vi "FV-resample-pad_data.vi"(11 "output cluster":T1) -> (1 "Array":cluster{"Y":dbl[], "Y":dbl[]}[](array[cluster]), 2 "appended array":waveform(dbl)[](array[waveform]), 3 "output cluster 2":T1)   [LabVIEW 2020, in "FV-file_viewer.lvlib"]
uses:
  FV-file_viewer.lvlib
  FV-splitting_data.ctl
  record_file_handler/VFH-file_cluster-R140.ctl
  record_file_handler/VFH-file_cluster-NanoVNA.ctl
  FV-water_cluster.ctl
  FV-single_XY_plot.ctl
  <vilib>/measure/maresamp.llb/Resample Waveform (single shot).vi
  <vilib>/measure/NI_MAPro.lvlib
  record_file_handler/VFH-VNA_File_Handler.lvlib
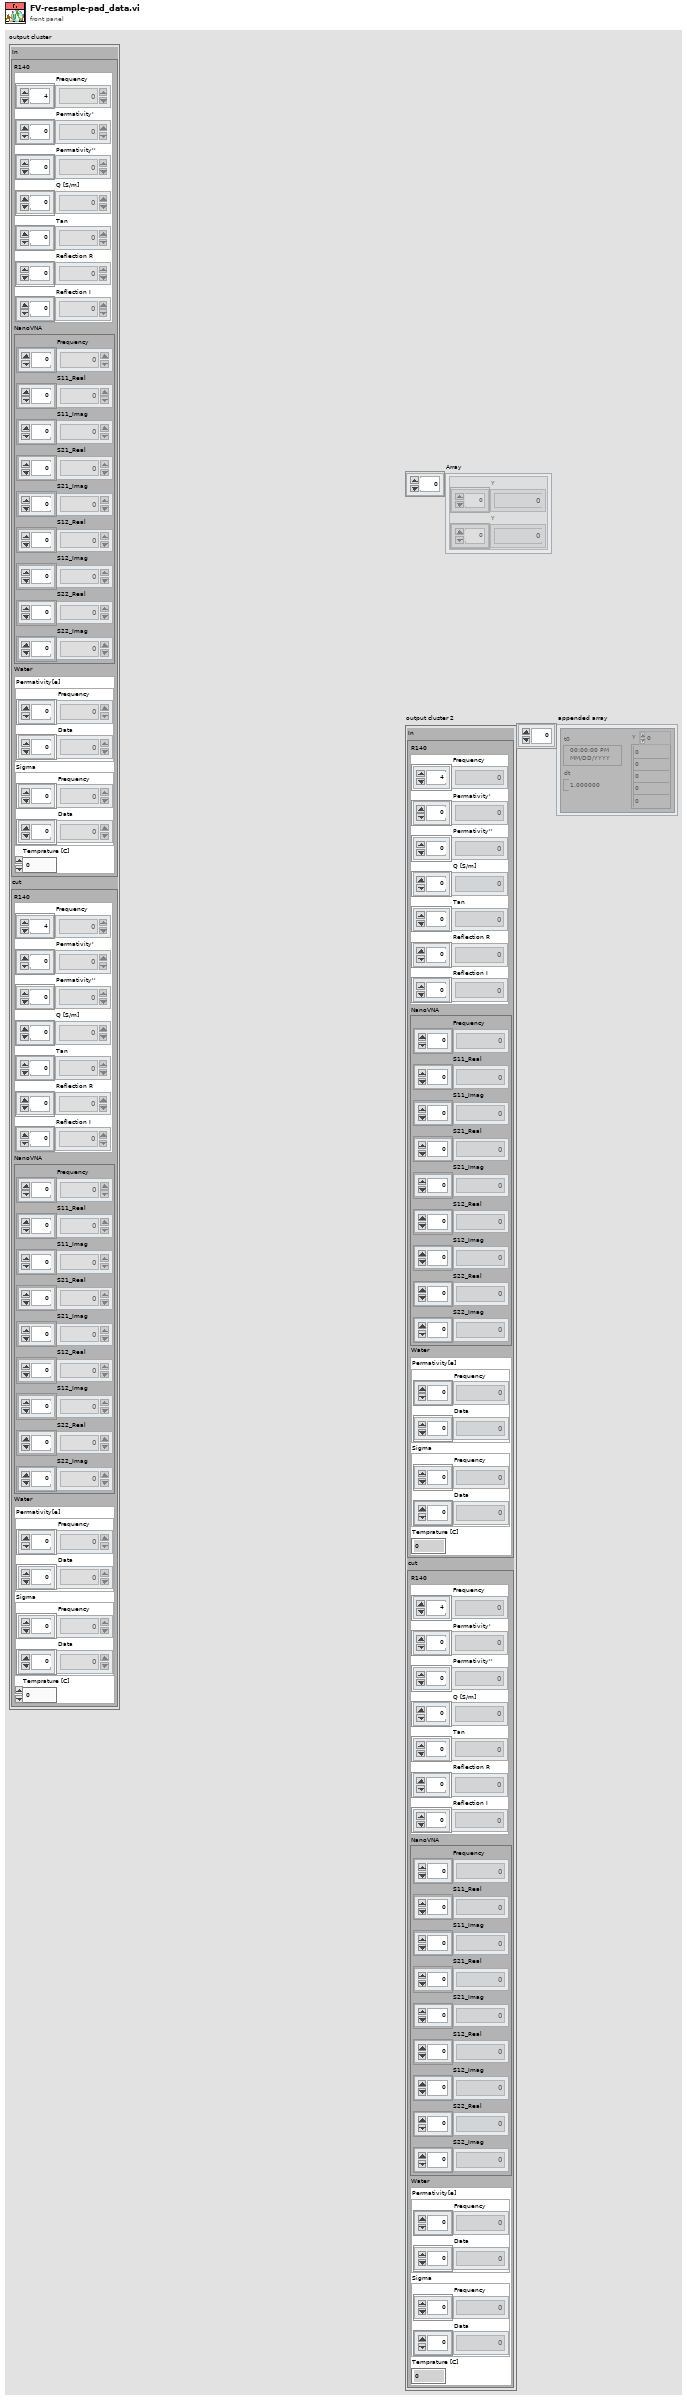
[diagram p1: front panel]
types:
  T1 = typedef "FV-file_viewer.lvlib/FV-splitting_data.ctl" = cluster{"In":cluster{"R140":T2, "NanoVNA":T3, "Water":T4}, "cut":cluster{"R140":T2, "NanoVNA":T3, "Water":T4}}
  T2 = typedef "VFH-VNA_File_Handler.lvlib/VFH-file_cluster-R140.ctl" = cluster{"Frequency":dbl[], "Permativity'":dbl[], "Permativity''":dbl[], "Q [S/m]":dbl[], "Tan":dbl[], "Reflection R":dbl[], "Reflection I":dbl[]}
  T3 = typedef "VFH-VNA_File_Handler.lvlib/VFH-file_cluster-NanoVNA.ctl" = cluster{"Frequency":dbl[], "S11_Real":dbl[], "S11_Imag":dbl[], "S21_Real":dbl[], "S21_Imag":dbl[], "S12_Real":dbl[], "S12_Imag":dbl[], "S22_Real":dbl[], "S22_Imag":dbl[]}
  T4 = typedef "FV-file_viewer.lvlib/FV-water_cluster.ctl" = cluster{"Permativity[e]":T5, "Sigma":T5, "Temprature [C]":dbl}
  T5 = typedef "FV-file_viewer.lvlib/FV-single_XY_plot.ctl" = cluster{"Frequency":dbl[], "Data":dbl[]}
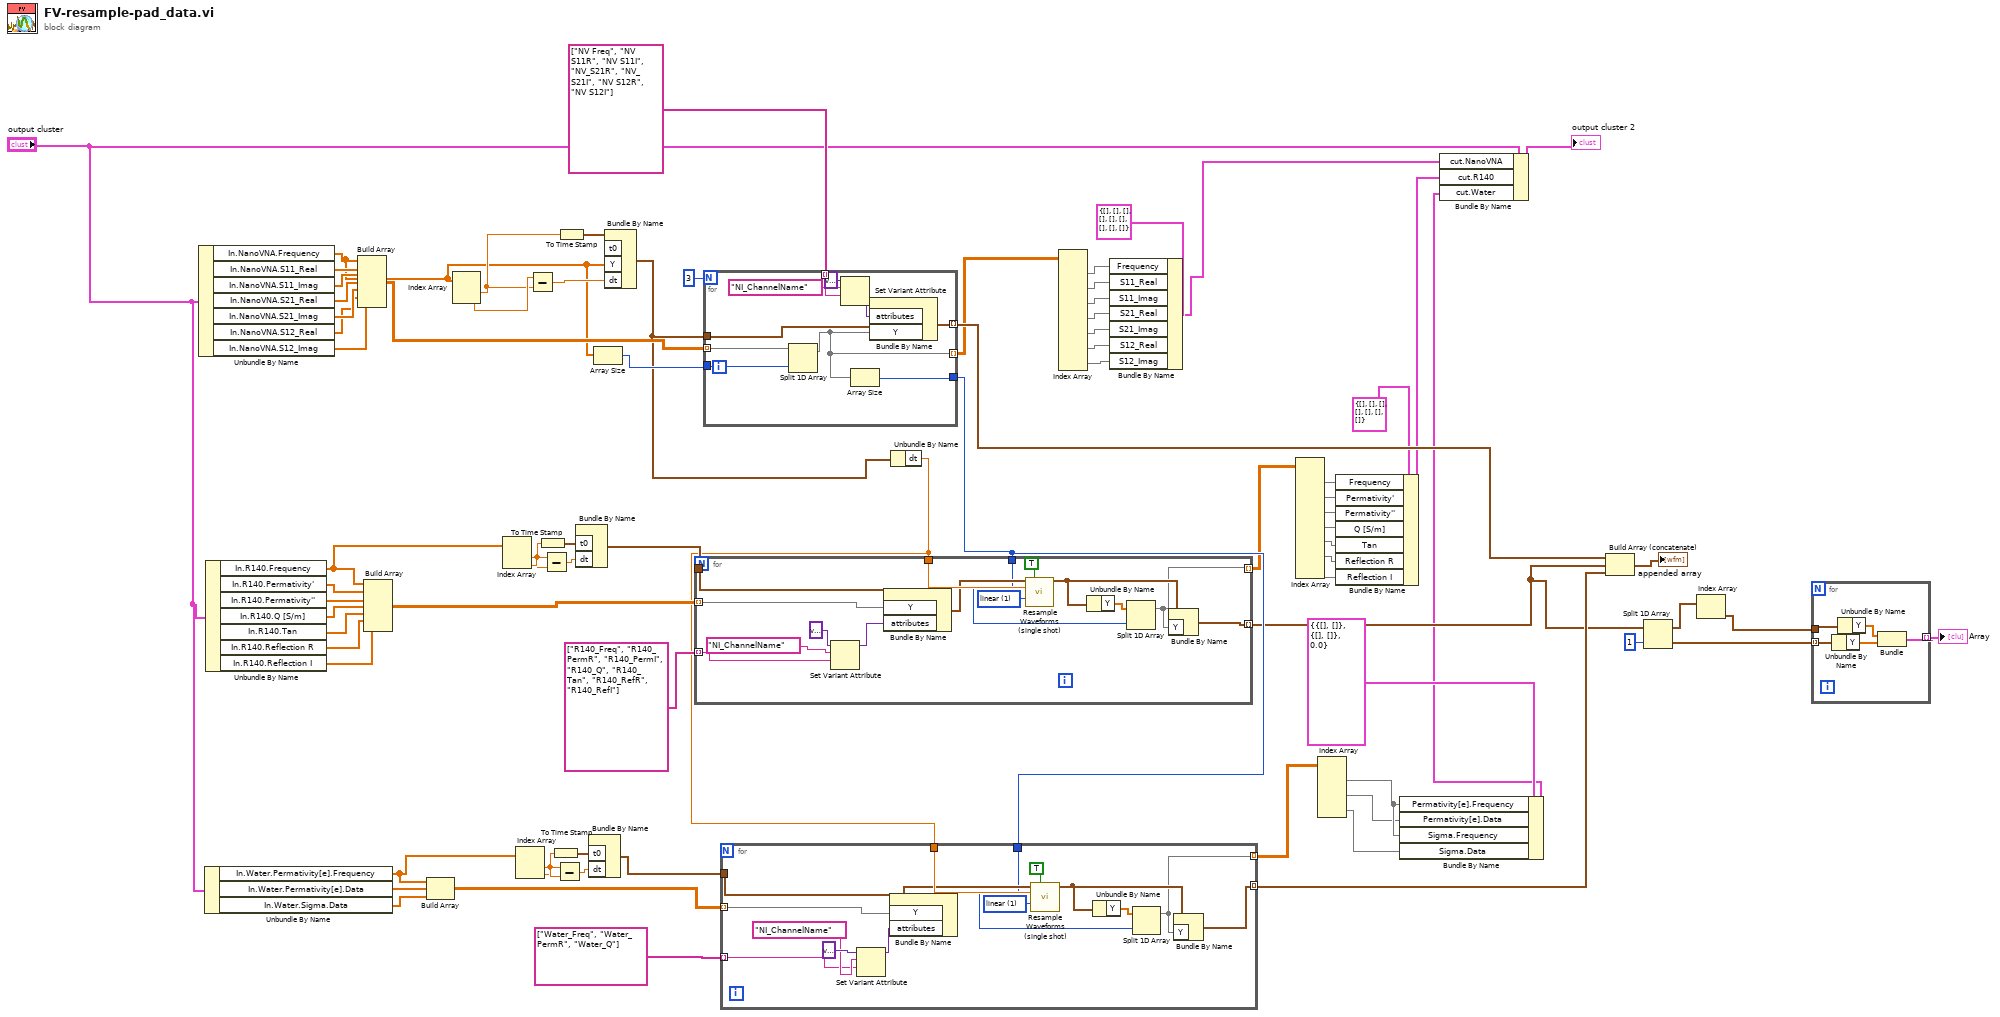
[diagram p0: block diagram]
diagram:
  n1 = Unbundle By Name("output cluster") -> ("In.NanoVNA.Frequency"=w54:dbl[], "In.NanoVNA.S11_Real"=w75:dbl[], "In.NanoVNA.S11_Imag"=w74:dbl[], "In.NanoVNA.S21_Real"=w73:dbl[], "In.NanoVNA.S21_Imag"=w72:dbl[], "In.NanoVNA.S12_Real"=w71:dbl[], "In.NanoVNA.S12_Imag"=w70:dbl[])
  n2 = Unbundle By Name("output cluster") -> ("In.Water.Permativity[e].Frequency"=w41:dbl[], "In.Water.Permativity[e].Data"=w52:dbl[], "In.Water.Sigma.Data"=w51:dbl[])
  n3 = Unbundle By Name("output cluster") -> ("In.R140.Frequency"=w63:dbl[], "In.R140.Permativity'"=w68:dbl[], "In.R140.Permativity''"=w67:dbl[], "In.R140.Q [S/m]"=w66:dbl[], "In.R140.Tan"=w65:dbl[], "In.R140.Reflection R"=w64:dbl[], "In.R140.Reflection I"=w48:dbl[])
  n4 = Build Array(w54, w75, w74, w73, w72, w71, w70) -> (w69:dbl[][])
  n5 = Build Array(w63, w68, w67, w66, w65, w64, w48) -> (w57:dbl[][])
  n6 = Build Array(w41, w52, w51) -> (w46:dbl[][])
  n7 = Index Array(array=w54) -> (element #1=w78:dbl, element #2=w79:dbl)  [unwired: 2 in]
  n8 = Index Array(array=w63) -> (element #1=w60:dbl, element #2=w62:dbl)  [unwired: 2 in]
  n9 = Index Array(array=w41) -> (element #1=w44:dbl, element #2=w42:dbl)  [unwired: 2 in]
  n10 = Subtract(x=w79, y=w78) -> (x-y=w76:dbl)
  n11 = To Time Stamp(1:w60) -> (0:w59:timestamp)
  n12 = Subtract(x=w62, y=w60) -> (x-y=w61:dbl)
  n13 = To Time Stamp(1:w44) -> (0:w45:timestamp)
  n14 = Subtract(x=w42, y=w44) -> (x-y=w43:dbl)
  n15 = To Time Stamp(1:w78) -> (0:w77:timestamp)
  n16 = Bundle By Name("t0"=w59, "dt"=w61) -> (w58:waveform(dbl))  [unwired: 1 in]
  n17 = Bundle By Name("t0"=w45, "dt"=w43) -> (w40:waveform(dbl))  [unwired: 1 in]
  n18 = Array Size(array=w54) -> (size(s)=w53:i32)
  n19 = Bundle By Name("t0"=w77, "Y"=w54, "dt"=w76) -> (w36:waveform(dbl))  [unwired: 1 in]
  n20 = for {
    N: 3 -> [_]
    tunnel: w36 -> [w89]
    tunnel: w69 -> [w86] mode=indexing
    tunnel: [w88] -> w56 mode=indexing
    tunnel: [w87] -> w38
    tunnel: w53 -> [w85]
    tunnel: string[] ["NV Freq", "NV S11R", "NV S11I", "NV_S21R", "NV_S21I", "NV S12R", "NV S12I"] ("name") -> [w82] mode=indexing
    tunnel: [w80] -> w33 mode=indexing
    n21 = Split 1D Array(array=w86, index=w85) -> (first subarray=w80:dbl[])  [unwired: 1 out]
    n22 = Set Variant Attribute(Variant=variant ("variant"), name="NI_ChannelName", value=w82) -> (Variant out=w84:variant)  [unwired: 1 in, 2 out]
    n23 = Array Size(array=w80) -> (size(s)=w87:i32)
    n24 = Bundle By Name(cluster=w89, "attributes"=w84, "Y"=w80) -> (w88:waveform(dbl))
  }
  n25 = Unbundle By Name(w36) -> ("dt"=w39:dbl)
  n26 = for {
    tunnel: w58 -> [w104]
    tunnel: w57 -> [w103] mode=indexing
    tunnel: w39 -> [w100]
    tunnel: [w95] -> w22 mode=indexing
    tunnel: w38 -> [w96]
    tunnel: string[] ["R140_Freq", "R140_PermR", "R140_PermI", "R140_Q", "R140_Tan", "R140_RefR", "R140_RefI"] ("name") -> [w91] mode=indexing
    tunnel: [w90] -> w15 mode=indexing
    w101 = u16 1 items=["coerce", "linear", "spline", "FIR filter"] ("interpolation mode")
    n27 = Set Variant Attribute(Variant=variant ("variant"), name="NI_ChannelName", value=w91) -> (Variant out=w94:variant)  [unwired: 1 in, 2 out]
    n28 = Bundle By Name(cluster=w104, "Y"=w103, "attributes"=w94) -> (w99:waveform(dbl))
    n29 = call-poly <vilib>:"Resample Waveforms (single shot).vi"("waveform in"=w99, "open interval? (F)"=TRUE, "dt"=w100, "interpolation mode"=w101) -> ("resampled waveform out"=w97:waveform(dbl))  [unwired: 8 in, 3 out]
    n30 = Unbundle By Name(w97) -> ("Y"=w98:dbl[])
    n31 = Split 1D Array(array=w98, index=w96) -> (first subarray=w90:dbl[])  [unwired: 1 out]
    n32 = Bundle By Name(cluster=w97, "Y"=w90) -> (w95:waveform(dbl))
  }
  n33 = for {
    tunnel: w40 -> [w119]
    tunnel: w46 -> [w118] mode=indexing
    tunnel: w39 -> [w115]
    tunnel: [w110] -> w37 mode=indexing
    tunnel: w38 -> [w111]
    tunnel: string[] ["Water_Freq", "Water_PermR", "Water_Q"] ("name") -> [w106] mode=indexing
    tunnel: [w105] -> w4 mode=indexing
    w116 = u16 1 items=["coerce", "linear", "spline", "FIR filter"] ("interpolation mode")
    n34 = Set Variant Attribute(Variant=variant ("variant"), name="NI_ChannelName", value=w106) -> (Variant out=w109:variant)  [unwired: 1 in, 2 out]
    n35 = Bundle By Name(cluster=w119, "Y"=w118, "attributes"=w109) -> (w114:waveform(dbl))
    n36 = call-poly <vilib>:"Resample Waveforms (single shot).vi"("waveform in"=w114, "open interval? (F)"=TRUE, "dt"=w115, "interpolation mode"=w116) -> ("resampled waveform out"=w112:waveform(dbl))  [unwired: 8 in, 3 out]
    n37 = Unbundle By Name(w112) -> ("Y"=w113:dbl[])
    n38 = Split 1D Array(array=w113, index=w111) -> (first subarray=w105:dbl[])  [unwired: 1 out]
    n39 = Bundle By Name(cluster=w112, "Y"=w105) -> (w110:waveform(dbl))
  }
  n40 = Index Array(array=w33) -> (element #1=w32:dbl[], element #2=w31:dbl[], element #3=w30:dbl[], element #4=w29:dbl[], element #5=w28:dbl[], element #6=w27:dbl[], element #7=w26:dbl[])  [unwired: 14 in]
  n41 = Bundle By Name(cluster=T3 {"Frequency"=[], "S11_Real"=[], "S11_Imag"=[], "S21_Real"=[], "S21_Imag"=[], "S12_Real"=[], "S12_Imag"=[], "S22_Real"=[], "S22_Imag"=[]} ("In.NanoVNA"), "Frequency"=w32, "S11_Real"=w31, "S11_Imag"=w30, "S21_Real"=w29, "S21_Imag"=w28, "S12_Real"=w27, "S12_Imag"=w26) -> (w24:T3)
  n42 = Index Array(array=w15) -> (element #1=w14:dbl[], element #2=w13:dbl[], element #3=w12:dbl[], element #4=w11:dbl[], element #5=w10:dbl[], element #6=w9:dbl[], element #7=w8:dbl[])  [unwired: 14 in]
  n43 = Index Array(array=w4) -> (element #1=w3:dbl[], element #2=w2:dbl[], element #3=w1:dbl[])  [unwired: 6 in]
  n44 = Bundle By Name(cluster=T2 {"Frequency"=[], "Permativity'"=[], "Permativity''"=[], "Q [S/m]"=[], "Tan"=[], "Reflection R"=[], "Reflection I"=[]} ("output cluster"), "Frequency"=w14, "Permativity'"=w13, "Permativity''"=w12, "Q [S/m]"=w11, "Tan"=w10, "Reflection R"=w9, "Reflection I"=w8) -> (w16:T2)
  n45 = Bundle By Name(cluster=T4 {"Permativity[e]"={"Frequency"=[], "Data"=[]}, "Sigma"={"Frequency"=[], "Data"=[]}, "Temprature [C]"=0.0} ("Water Raw"), "Permativity[e].Frequency"=w3, "Permativity[e].Data"=w2, "Sigma.Frequency"=w3, "Sigma.Data"=w1) -> (w5:T4)
  n46 = Bundle By Name(cluster="output cluster", "cut.NanoVNA"=w24, "cut.R140"=w16, "cut.Water"=w5) -> (→"output cluster 2":T1)
  n47 = Build Array (concatenate)(w56, w22, w37) -> (→"appended array":waveform(dbl)[])
  n48 = Split 1D Array(array=w22, index=1) -> (first subarray=w20:waveform(dbl)[], second subarray=w18:waveform(dbl)[])
  n49 = Index Array(array=w20) -> (element=w19:waveform(dbl))  [unwired: 1 in]
  n50 = for {
    tunnel: w19 -> [w124]
    tunnel: w18 -> [w123] mode=indexing
    tunnel: [w120] -> w17 mode=indexing
    n51 = Unbundle By Name(w123) -> ("Y"=w122:dbl[])
    n52 = Unbundle By Name(w124) -> ("Y"=w121:dbl[])
    n53 = Bundle("Y"=w121, "Y"=w122) -> (w120:cluster{"Y":dbl[], "Y":dbl[]})  [unwired: 1 in]
  }
  "Array" <- w17
